vi "OpenDAQmxDevice.vi"(8 "error in":errorcluster) -> (0 "error out":errorcluster, 2 "physical channel":tag[](array[tag])=["cDAQ1Mod1/ao0", "cDAQ1Mod1/ao1", "cDAQ1Mod1/ao2", "cDAQ1Mod1/ao3", "cDAQ1Mod1/ao4", "cDAQ1Mod1/ao5", "cDAQ1Mod1/ao6", "cDAQ1Mod1/ao7", "cDAQ1Mod1/ao8", "cDAQ1Mod1/ao9", "cDAQ1Mod1/ao10", "cDAQ1Mod1/ao11", "cDAQ1Mod1/ao12", "cDAQ1Mod1/ao13", "cDAQ1Mod1/ao14", "cDAQ1Mod1/ao15"], 3 "task out":refnum<k21>)   [LabVIEW 2014]
uses:
  <vilib>/DAQmx/create/channels.llb/DAQmx Create Channel (AO-Voltage-Basic).vi
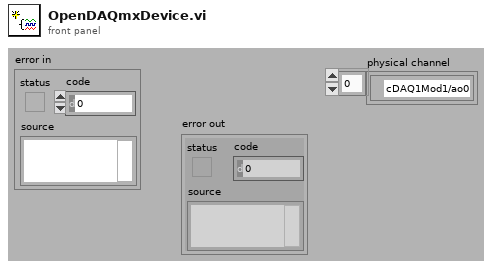
[diagram p1: front panel]
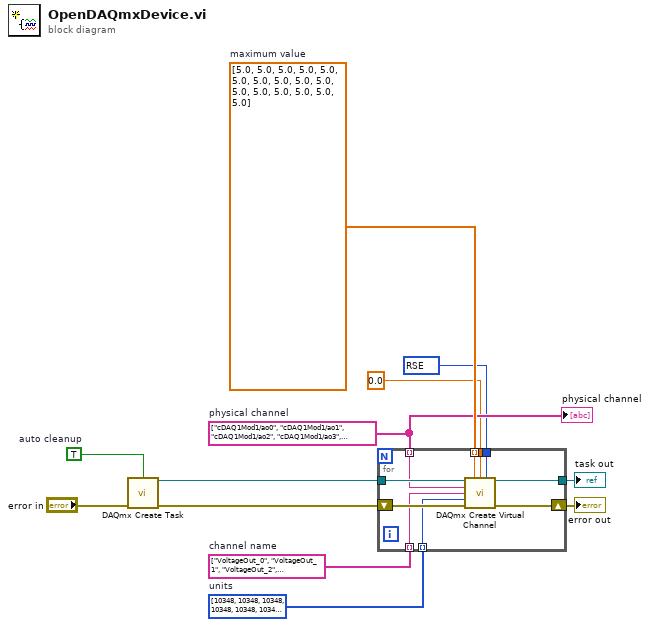
[diagram p0: block diagram]
diagram:
  w2 = 10083 items=["Default"=-1, "RSE"=10083, "Differential"=10106, "Pseudodifferential"=12529] ("output terminal configuration")
  w7 = i32[] [10348, 10348, 10348, 10348, 10348, 10348, 10348, 10348, 10348, 10348, 10348, 10348, 10348, 10348, 10348, 10348] items=["Volts"=10348, "From Custom Scale"=10065]  # units
  w6 = string[] ["VoltageOut_0", "VoltageOut_1", "VoltageOut_2", "VoltageOut_3", "VoltageOut_4", "VoltageOut_5", "VoltageOut_6", "VoltageOut_7", "VoltageOut_8", "VoltageOut_9", "VoltageOut_10", "VoltageOut_11", "VoltageOut_12", "VoltageOut_13", "VoltageOut_14", "VoltageOut_15"]  # channel name
  w5 = tag[] ["cDAQ1Mod1/ao0", "cDAQ1Mod1/ao1", "cDAQ1Mod1/ao2", "cDAQ1Mod1/ao3", "cDAQ1Mod1/ao4", "cDAQ1Mod1/ao5", "cDAQ1Mod1/ao6", "cDAQ1Mod1/ao7", "cDAQ1Mod1/ao8", "cDAQ1Mod1/ao9", "cDAQ1Mod1/ao10", "cDAQ1Mod1/ao11", "cDAQ1Mod1/ao12", "cDAQ1Mod1/ao13", "cDAQ1Mod1/ao14", "cDAQ1Mod1/ao15"]  # physical channel
  w8 = dbl[] [5.0, 5.0, 5.0, 5.0, 5.0, 5.0, 5.0, 5.0, 5.0, 5.0, 5.0, 5.0, 5.0, 5.0, 5.0, 5.0]  # maximum value
  w10 = TRUE  # auto cleanup
  n1 = call <vilib>:"DAQmx Create Task.vi"("auto cleanup"=w10, "error in"="error in") -> ("task out"=w9:refnum<k21>, "error out"=w11:errorcluster)  [unwired: 12 in]
  n2 = for {
    tunnel: w9 -> [w20]
    tunnel: 0.0 ("minimum value") -> [w21]
    tunnel: w8 -> [w22] mode=indexing
    tunnel: w7 -> [w15] mode=indexing
    tunnel: w6 -> [w16] mode=indexing
    tunnel: w5 -> [w13] mode=indexing
    tunnel: [w18] -> w4
    shift-right: [w17] -> w3
    shift-left: w11 -> [w19]
    tunnel: w2 -> [w14]
    n3 = call-poly <vilib>:"DAQmx Create Virtual Channel.vi"("task in"=w20, "maximum value"=w22, "minimum value"=w21, "output terminal configuration"=w14, "physical channels"=w13, "name to assign"=w16, "units"=w15, "error in"=w19) -> ("task out"=w18:refnum<k21>, "error out"=w17:errorcluster)  [unwired: 6 in]
  }
  "error out" <- w3
  "task out" <- w4
  "physical channel" <- w5
